vi "Init.vi"(4 "CS Active Low (T)":bool=TRUE, 5 "CS GPIO (None)":T1=-1, 7 "SPI #":T2=-1, 8 "error in (no error)":errorcluster) -> (0 "error out":errorcluster, 3 "SPI Device out":refnum<class "SPI Peripheral.lvclass">)   [LabVIEW 2020, in "CTI.lvlib" / "SPI Peripheral.lvclass"]
uses:
  SPI Peripheral.lvclass
  SPI Number.ctl
  GPIO Number.ctl
  SPI Peripheral.lvclass/SPI Peripheral.ctl
  CTI.lvlib
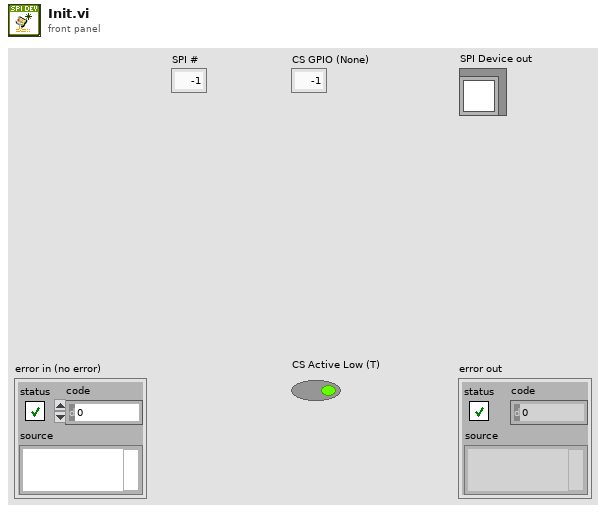
[diagram p1: front panel]
types:
  T1 = typedef "CTI.lvlib/GPIO Number.ctl" = i8
  T2 = typedef "CTI.lvlib/SPI Number.ctl" = i8
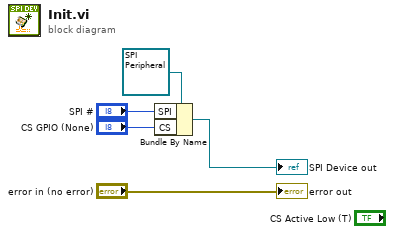
[diagram p0: block diagram]
diagram:
  n1 = Bundle By Name(cluster=refnum<class "SPI Peripheral.lvclass"> refnum ("SPI Device in"), "SPI"="SPI #", "CS"="CS GPIO (None)") -> (→"SPI Device out":refnum<class "SPI Peripheral.lvclass">)
  "error out" <- "error in (no error)"
